vi "Configure Trigger Mode.vi"(0 "VISA resource name":refnum<visa-resource-name>, 1 "Trigger Holdoff (1E-7 s)":dbl=1e-07, 5 "Trigger Mode (2: Edge)":i32(ring)=2 items=["Communication", "Delay", "Edge ", "Glitch", "Pattern", "Pulse Width ", "Runt", "Setup and Hold Time", "State", "Timeout", "Transition", "TV", "Window", "Advanced", "Serial Bus 1", "Serial Bus 2", "Serial Bus 3", "Serial Bus 4"], 11 "error in (no error)":errorcluster) -> (4 "VISA resource name out":refnum<visa-resource-name>, 15 "error out":errorcluster)   [LabVIEW 2020, in "Agilent 90000 Series.lvlib"]
doc: "Configures the trigger mode of an oscilloscope."
uses:
  Agilent 90000 Series.lvlib
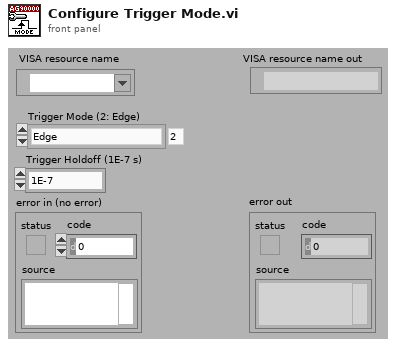
[diagram p1: front panel]
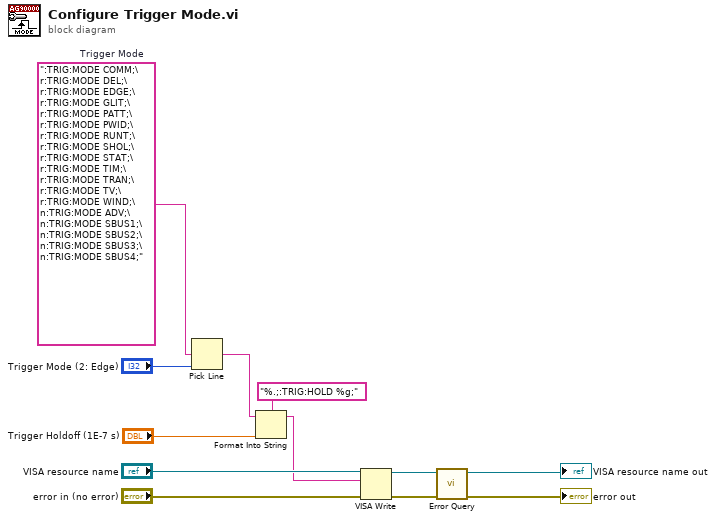
[diagram p0: block diagram]
diagram:
  w12 = ":TRIG:MODE COMM;\r:TRIG:MODE DEL;\r:TRIG:MODE EDGE;\r:TRIG:MODE GLIT;\r:TRIG:MODE PATT;\r:TRIG:MODE PWID;\r:TRIG:MODE RUNT;\r:TRIG:MODE SHOL;\r:TRIG:MODE STAT;\r:TRIG:MODE TIM;\r:TRIG:MODE TRAN;\r:TRIG:MODE TV;\r:TRIG:MODE WIND;\n:TRIG:MODE ADV;\n:TRIG:MODE SBUS1;\n:TRIG:MODE SBUS2;\n:TRIG:MODE SBUS3;\n:TRIG:MODE SBUS4;"  # Trigger Mode
  n1 = Pick Line(multi-line string=w12, line index="Trigger Mode (2: Edge)") -> (output string=w1:string)  [unwired: 1 out]
  n2 = Format Into String(format string="%.;:TRIG:HOLD %g;", initial string=w1, "Trigger Holdoff (1E-7 s)") -> (resulting string=w4:string)  [unwired: 1 in, 1 out]
  n3 = VISA Write(VISA resource name="VISA resource name", write buffer=w4, error in (no error)="error in (no error)") -> (VISA resource name out=w8:refnum<visa-resource-name>, error out=w7:errorcluster)  [unwired: 1 out]
  n4 = call "Error Query.vi"("error in (no error)"=w7, "VISA resource name"=w8) -> ("error out"=→"error out":errorcluster, "VISA resource name out"=→"VISA resource name out":refnum<visa-resource-name>)  [unwired: 8 out]
